vi "IDE_BT_Example.vi"() -> ()   [LabVIEW 2020]
uses:
  Subs/ColorText/Code.xctl
  Subs/Console XCtrl/Console_Xctrl.xctl
  Subs/Server XCtrl/Server.xctl
panel:
  in  "Files 2":bool
  in  "Open Server 2":bool
  in  "Help 2":bool
  in  "Name 2":string="code.py"
  in  "Save 2":bool
  in  "Stop 2":bool
  in  "Pyboard":string(xcontrol)="\n'''\nmac address of pybd: b'HJ0\\x01o\\xf2' or 48:4A:01:6F:F2\n    '''\n    '''\nHR_UUID = ubluetooth.UUID(0x180D)\nHR_CHAR = (ubluetooth.UUID(0x2A37), ubluetooth.FLAG_READ | ubluetooth.FLAG_NOTIFY,)\nHR_SERVICE = (HR_UUID, (HR_CHAR,),)\nSERVICES = (HR_SERVICE, )\n(hr,) = bt.gatts_register_services(SERVICES)\n'''\n\nimport bluetooth,utime\n\nble = bluetooth.BLE()\nble.active(True)\n\nLWP_CHAR = (\n    bluetooth.UUID('00001624-1212-EFDE-1623-785FEABCD123'),\n    bluetooth.FLAG_WRITE | bluetooth.FLAG_NOTIFY,\n    # List of descriptors\n    (\n        # CCCD\n        (bluetooth.UUID(0x2902), bluetooth.FLAG_READ | bluetooth.FLAG_WRITE),\n    )\n)\nLPF2_SERVICE = (bluetooth.UUID('03971101-0000-1000-8000-00805F9B34FB'), (LWP_CHAR,))\nALL_SERVICES = (LPF2_SERVICE,)\n\n(lwp_char, lwp_descr), = ble.gatts_register_services(ALL_SERVICES)\n\ndef bt_irq(x, y):\n    print('bt_irq', x, y)\n    \nble.irq(bt_irq)\n\ndef adv_encode_name(name):\n    name = bytes(name, 'ascii')\n    return bytearray((len(name) + 1, 0x09)) + name\n    \ndef adv(name):\n    ble.gap_advertise(100_000, adv_data=b'\\x02\\x01\\x06' + adv_encode_name(name))\n    \nadv('pybd-lpf2')\n\nutime.sleep(5)   # wait for pyboard to get ready and connect\n\nble.gatts_notify(64, lwp_char, 'from pybd')\n\nble.gatts_read(lwp_char)\n"
  in  "Run 2":bool
  in  "Clean 2":bool
  in  "PC Save 2":bool
  in  "PC path 2":path
  in  "Clear 2":bool
  out "REPL 2":string(xcontrol)="bt_irq', event, data)\n... \n... bt.irq(bt_irq, bluetooth.IRQ_ALL)\n... '''\n\"\\ndef bt_irq(event, data):\\n    print('bt_irq', event, data)\\n\\nbt.irq(bt_irq, bluetooth.IRQ_ALL)\\n\"\n>>> blurtooth.\nTraceback (most recent call last):\n  File \"<stdin>\", line 2\nSyntaxError: invalid syntax\n>>> bluetooth.\n__class__       __name__        BLE             FLAG_NOTIFY\nFLAG_READ       FLAG_WRITE      UUID\n>>> bt.\n__class__       active          config          gap_advertise\ngap_connect     gap_disconnect  gap_scan\ngattc_discover_characteristics  gattc_discover_descriptors\ngattc_discover_services         gattc_read      gattc_write\ngatts_notify    gatts_read      gatts_register_services\ngatts_set_buffer                gatts_write     irq\n>>> import bluetooth\n>>> bt = bluetooth.BLE()\n>>> bt.active(True)\nTrue\n>>> LPF2_SERVICE = bluetooth.UUID('00001623-1212-EFDE-1623-785FEABCD123')\n>>> LWP_CHAR = (bluetooth.UUID('00001624-1212-EFDE-1623-785FEABCD123'), bluetooth.FLAG_NOTIFY|bluetooth.FLAG_WRITE,)\n>>> lwp_char, = bt.gatts_register_services(LPF2_SERVICE, (LWP_CHAR,))\nTraceback (most recent call last):\n  File \"<stdin>\", line 1, in <module>\nTypeError: function takes 2 positional arguments but 3 were given\n>>> bt.gap_advertise(100, adv_data=bytearray('\\x02\\x01\\x02\\x0a\\x09pybd-lpf2'))\n>>> bt.gatts_notify(lwp_char, 64, 'from pybd')\nTraceback (most recent call last):\n  File \"<stdin>\", line 1, in <module>\nNameError: name 'lwp_char' isn't defined\n>>> bt.gatts_read(lwp_char)\nTraceback (most recent call last):\n  File \"<stdin>\", line 1, in <module>\nNameError: name 'lwp_char' isn't defined\n>>> '''\n... def bt_irq(event, data):\n...     print('bt_irq', event, data)\n... \n... bt.irq(bt_irq, bluetooth.IRQ_ALL)\n... '''\n\"\\ndef bt_irq(event, data):\\n    print('bt_irq', event, data)\\n\\nbt.irq(bt_irq, bluetooth.IRQ_ALL)\\n\"\n>>> '''\n... mac address of pybd: b'HJ0\\x01o\\xf2' or 48:4A:01:6F:F2\n... '''\n\"\\nmac address of pybd: b'HJ0\\x01o\\xf2' or 48:4A:01:6F:F2\\n\"\n>>> '''\n... \n... HR_UUID = ubluetooth.UUID(0x180D)\n... HR_CHAR = (ubluetooth.UUID(0x2A37), ubluetooth.FLAG_READ | ubluetooth.FLAG_NOTIFY,)\n... HR_SERVICE = (HR_UUID, (HR_CHAR,),)\n... SERVICES = (HR_SERVICE, )\n... (hr,) = bt.gatts_register_services(SERVICES)\n... '''\n'\\n\\nHR_UUID = ubluetooth.UUID(0x180D)\\nHR_CHAR = (ubluetooth.UUID(0x2A37), ubluetooth.FLAG_READ | ubluetooth.FLAG_NOTIFY,)\\nHR_SERVICE = (HR_UUID, (HR_CHAR,),)\\nSERVICES = (HR_SERVICE, )\\n(hr,) = bt.gatts_register_services(SERVICES)\\n'\n>>> import bluetooth,utime\n>>> ble = bluetooth.BLE()\n>>> ble.active(True)\nTrue\n>>> LWP_CHAR = (\n... bluetooth.UUID('00001624-1212-EFDE-1623-785FEABCD123'),\n... bluetooth.FLAG_WRITE | bluetooth.FLAG_NOTIFY,\n... (\n... (bluetooth.UUID(0x2902), bluetooth.FLAG_READ | bluetooth.FLAG_WRITE),\n... )\n... \n... )\n>>> LPF2_SERVICE = (bluetooth.UUID('00001623-1212-EFDE-1623-785FEABCD123'), (LWP_CHAR,))\n>>> ALL_SERVICES = (LPF2_SERVICE,)\n>>> (lwp_char, lwp_descr), = ble.gatts_register_services(ALL_SERVICES)\n>>> def bt_irq(x, y):\n...     print('bt_irq', x, y)\n... \n>>> ble.irq(bt_irq)\n>>> def adv_encode_name(name):\n...     name = bytes(name, 'ascii')\n...     return bytearray((len(name) + 1, 0x09)) + name\n... \n>>> def adv(name):\n...     ble.gap_advertise(100_000, adv_data=b'\\x02\\x01\\x06' + adv_encode_name(name))\n... \n>>> adv('pybd-lpf2')\n>>> utime.sleep(5)   \n>>> ble.gatts_notify(64, lwp_char, 'from pybd')\nTraceback (most recent call last):\n  File \"<stdin>\", line 1, in <module>\nOSError: [Errno 107] ENOTCONN\n>>> ble.gatts_read(lwp_char)\nb''\n>>> '''\n... mac address of pybd: b'HJ0\\x01o\\xf2' or 48:4A:01:6F:F2\n... '''\n\"\\nmac address of pybd: b'HJ0\\x01o\\xf2' or 48:4A:01:6F:F2\\n\"\n>>> '''\n... \n... HR_UUID = ubluetooth.UUID(0x180D)\n... HR_CHAR = (ubluetooth.UUID(0x2A37), ubluetooth.FLAG_READ | ubluetooth.FLAG_NOTIFY,)\n... HR_SERVICE = (HR_UUID, (HR_CHAR,),)\n... SERVICES = (HR_SERVICE, )\n... (hr,) = bt.gatts_register_services(SERVICES)\n... '''\n'\\n\\nHR_UUID = ubluetooth.UUID(0x180D)\\nHR_CHAR = (ubluetooth.UUID(0x2A37), ubluetooth.FLAG_READ | ubluetooth.FLAG_NOTIFY,)\\nHR_SERVICE = (HR_UUID, (HR_CHAR,),)\\nSERVICES = (HR_SERVICE, )\\n(hr,) = bt.gatts_register_services(SERVICES)\\n'\n>>> import bluetooth,utime\n>>> ble = bluetooth.BLE()\n>>> ble.active(True)\nTrue\n>>> LWP_CHAR = (\n... bluetooth.UUID('00001624-1212-EFDE-1623-785FEABCD123'),\n... bluetooth.FLAG_WRITE | bluetooth.FLAG_NOTIFY,\n... (\n... (bluetooth.UUID(0x2902), bluetooth.FLAG_READ | bluetooth.FLAG_WRITE),\n... )\n... \n... )\n>>> LPF2_SERVICE = (bluetooth.UUID('00001623-1212-EFDE-1623-785FEABCD123'), (LWP_CHAR,))\n>>> ALL_SERVICES = (LPF2_SERVICE,)\n>>> (lwp_char, lwp_descr), = ble.gatts_register_services(ALL_SERVICES)\n>>> def bt_irq(x, y):\n...     print('bt_irq', x, y)\n... \n>>> ble.irq(bt_irq)\n>>> def adv_encode_name(name):\n...     name = bytes(name, 'ascii')\n...     return bytearray((len(name) + 1, 0x09)) + name\n... \n>>> def adv(name):\n...     ble.gap_advertise(100_000, adv_data=b'\\x02\\x01\\x06' + adv_encode_name(name))\n... \n>>> adv('pybd-lpf2')\n>>> utime.sleep(5)   \n>>> ble.gatts_notify(64, lwp_char, 'from pybd')\nTraceback (most recent call last):\n  File \"<stdin>\", line 1, in <module>\nOSError: [Errno 107] ENOTCONN\n>>> ble.gatts_read(lwp_char)\nb''\n>>> '''\n... mac address of pybd: b'HJ0\\x01o\\xf2' or 48:4A:01:6F:F2\n... '''\n\"\\nmac address of pybd: b'HJ0\\x01o\\xf2' or 48:4A:01:6F:F2\\n\"\n>>> '''\n... \n... HR_UUID = ubluetooth.UUID(0x180D)\n... HR_CHAR = (ubluetooth.UUID(0x2A37), ubluetooth.FLAG_READ | ubluetooth.FLAG_NOTIFY,)\n... HR_SERVICE = (HR_UUID, (HR_CHAR,),)\n... SERVICES = (HR_SERVICE, )\n... (hr,) = bt.gatts_register_services(SERVICES)\n... '''\n'\\n\\nHR_UUID = ubluetooth.UUID(0x180D)\\nHR_CHAR = (ubluetooth.UUID(0x2A37), ubluetooth.FLAG_READ | ubluetooth.FLAG_NOTIFY,)\\nHR_SERVICE = (HR_UUID, (HR_CHAR,),)\\nSERVICES = (HR_SERVICE, )\\n(hr,) = bt.gatts_register_services(SERVICES)\\n'\n>>> import bluetooth,utime\n>>> ble = bluetooth.BLE()\n>>> ble.active(True)\nTrue\n>>> LWP_CHAR = (\n... bluetooth.UUID('00001624-1212-EFDE-1623-785FEABCD123'),\n... bluetooth.FLAG_WRITE | bluetooth.FLAG_NOTIFY,\n... (\n... (bluetooth.UUID(0x2902), bluetooth.FLAG_READ | bluetooth.FLAG_WRITE),\n... )\n... \n... )\n>>> LPF2_SERVICE = (bluetooth.UUID('03971101-0000-1000-8000-00805F9B34FB'), (LWP_CHAR,))\n>>> ALL_SERVICES = (LPF2_SERVICE,)\n>>> (lwp_char, lwp_descr), = ble.gatts_register_services(ALL_SERVICES)\n>>> def bt_irq(x, y):\n...     print('bt_irq', x, y)\n... \n>>> ble.irq(bt_irq)\n>>> def adv_encode_name(name):\n...     name = bytes(name, 'ascii')\n...     return bytearray((len(name) + 1, 0x09)) + name\n... \n>>> def adv(name):\n...     ble.gap_advertise(100_000, adv_data=b'\\x02\\x01\\x06' + adv_encode_name(name))\n... \n>>> adv('pybd-lpf2')\n>>> utime.sleep(5)   \n>>> ble.gatts_notify(64, lwp_char, 'from pybd')\nTraceback (most recent call last):\n  File \"<stdin>\", line 1, in <module>\nOSError: [Errno 107] ENOTCONN\n>>> ble.gatts_read(lwp_char)\nb''\n>>> \nMPY: sync filesystems\nMPY: soft reboot\nMicroPython v1.11-611-g7f24c2977-dirty on 2019-11-29; PYBD-SF2W with STM32F722IEK\nType \"help()\" for more information.\n>>> '''\n... mac address of pybd: b'HJ0\\x01o\\xf2' or 48:4A:01:6F:F2\n... '''\n\"\\nmac address of pybd: b'HJ0\\x01o\\xf2' or 48:4A:01:6F:F2\\n\"\n>>> '''\n... \n... HR_UUID = ubluetooth.UUID(0x180D)\n... HR_CHAR = (ubluetooth.UUID(0x2A37), ubluetooth.FLAG_READ | ubluetooth.FLAG_NOTIFY,)\n... HR_SERVICE = (HR_UUID, (HR_CHAR,),)\n... SERVICES = (HR_SERVICE, )\n... (hr,) = bt.gatts_register_services(SERVICES)\n... '''\n'\\n\\nHR_UUID = ubluetooth.UUID(0x180D)\\nHR_CHAR = (ubluetooth.UUID(0x2A37), ubluetooth.FLAG_READ | ubluetooth.FLAG_NOTIFY,)\\nHR_SERVICE = (HR_UUID, (HR_CHAR,),)\\nSERVICES = (HR_SERVICE, )\\n(hr,) = bt.gatts_register_services(SERVICES)\\n'\n>>> import bluetooth,utime\n>>> ble = bluetooth.BLE()\n>>> ble.active(True)\nTrue\n>>> LWP_CHAR = (\n... bluetooth.UUID('00001624-1212-EFDE-1623-785FEABCD123'),\n... bluetooth.FLAG_WRITE | bluetooth.FLAG_NOTIFY,\n... (\n... (bluetooth.UUID(0x2902), bluetooth.FLAG_READ | bluetooth.FLAG_WRITE),\n... )\n... \n... )\n>>> LPF2_SERVICE = (bluetooth.UUID('03971101-0000-1000-8000-00805F9B34FB'), (LWP_CHAR,))\n>>> ALL_SERVICES = (LPF2_SERVICE,)\n>>> (lwp_char, lwp_descr), = ble.gatts_register_services(ALL_SERVICES)\n>>> def bt_irq(x, y):\n...     print('bt_irq', x, y)\n... \n>>> ble.irq(bt_irq)\n>>> def adv_encode_name(name):\n...     name = bytes(name, 'ascii')\n...     return bytearray((len(name) + 1, 0x09)) + name\n... \n>>> def adv(name):\n...     ble.gap_advertise(100_000, adv_data=b'\\x02\\x01\\x06' + adv_encode_name(name))\n... \n>>> adv('pybd-lpf2')\n>>> utime.sleep(5)   \n>>> ble.gatts_notify(64, lwp_char, 'from pybd')\nTraceback (most recent call last):\n  File \"<stdin>\", line 1, in <module>\nOSError: [Errno 107] ENOTCONN\n>>> ble.gatts_read(lwp_char)\nb''\n>>> bt_irq 1 (64, 1, b\"N'\\xee\\xa63)\")\nbt_irq 4 (64, 13)\nbt_irq 4 (64, 13)\n\n>>> ble.gatts_read(lwp_char)\nb'\\xff'\n>>> bt_irq 4 (64, 13)\n\n>>> ble.gatts_read(lwp_char)\nb'z'\n>>> ble.\n__class__       active          config          gap_advertise\ngap_connect     gap_disconnect  gap_scan\ngattc_discover_characteristics  gattc_discover_descriptors\ngattc_discover_services         gattc_read      gattc_write\ngatts_notify    gatts_read      gatts_register_services\ngatts_set_buffer                gatts_write     irq\n>>> bluetooth.\n__class__       __name__        BLE             FLAG_NOTIFY\nFLAG_READ       FLAG_WRITE      UUID\n>>> bluetooth.UUID()\nTraceback (most recent call last):\n  File \"<stdin>\", line 1, in <module>\nTypeError: function takes 1 positional arguments but 0 were given\n>>> \n>>> bt_irq 2 (64, 1, b\"N'\\xee\\xa63)\")\n\n>>> bluetooth.\n__class__       __name__        BLE             FLAG_NOTIFY\nFLAG_READ       FLAG_WRITE      UUID\n>>> bluetooth.BLE.\n__class__       __name__        __bases__       active\nconfig          gap_advertise   gap_connect     gap_disconnect\ngap_scan        gattc_discover_characteristics\ngattc_discover_descriptors      gattc_discover_services\ngattc_read      gattc_write     gatts_notify    gatts_read\ngatts_register_services         gatts_set_buffer\ngatts_write     irq\n>>> bluetooth.BLE."
  in  "Server 2":path(xcontrol)=path "/Users/crogers/GitHub/Summer2020/LabVIEWCode/Servers/Damien.vi"
  in  "Clean":bool
  in  "PC Save":bool
  in  "PC path":path
  in  "Files":bool
  in  "Open Server":bool
  in  "Help":bool
  in  "Server":path(xcontrol)=path "/Users/crogers/GitHub/Summer2020/LabVIEWCode/Servers/Jens.vi"
  out "REPL":string(xcontrol)="p\":[[0, []], [0, []], [0, []], [0, []], [0, []], [0, []], [-31, 30, 995], [2, 5, 1], [8, 1, -1], \"\", 0]}{\"m\":0,\"p\":[[0, []], [0, []], [0, []], [0, []], [0, []], [0, []], [-30, 27, 991], [3, 5, 1], [8, 1, -1], \"\", 0]}{\"m\":0,\"p\":[[0, []], [0, []], [0, []], [0, []], [0, []], [0, []], [-29, 26, 993], [2, 5, 1], [8, 1, -1], \"\", 0]}{\"m\":0,\"p\":[[0, []], [0, []], [0, []], [0, []], [0, []], [0, []], [-29, 28, 992], [3, 5, 0], [8, 1, -1], \"\", 0]}{\"m\":0,\"p\":[[0, []], [0, []], [0, []], [0, []], [0, []], [0, []], [-29, 28, 990], [3, 5, 1], [8, 1, -1], \"\", 0]}{\"m\":0,\"p\":[[0, []], [0, []], [0, []], [0, []], [0, []], [0, []], [-29, 27, 994], [2, 5, 1], [8, 1, -1], \"\", 0]}{\"m\":0,\"p\":[[0, []], [0, []], [0, []], [0, []], [0, []], [0, []], [-29, 30, 991], [3, 5, 1], [8, 1, -1], \"\", 0]}{\"m\":0,\"p\":[[0, []], [0, []], [0, []], [0, []], [0, []], [0, []], [-27, 27, 993], [3, 5, 1], [8, 1, -1], \"\", 0]}{\"m\":0,\"p\":[[0, []], [0, []], [0, []], [0, []], [0, []], [0, []], [-29, 28, 992], [2, 4, 1], [8, 1, -1], \"\", 0]}{\"m\":0,\"p\":[[0, []], [0, []], [0, []], [0, []], [0, []], [0, []], [-29, 28, 989], [2, 5, 1], [8, 1, -1], \"\", 0]}{\"m\":0,\"p\":[[0, []], [0, []], [0, []], [0, []], [0, []], [0, []], [-28, 28, 989], [2, 5, 1], [8, 1, -1], \"\", 0]}{\"m\":0,\"p\":[[0, []], [0, []], [0, []], [0, []], [0, []], [0, []], [-28, 29, 992], [3, 5, 1], [8, 1, -1], \"\", 0]}{\"m\":0,\"p\":[[0, []], [0, []], [0, []], [0, []], [0, []], [0, []], [-28, 28, 993], [3, 5, 0], [8, 1, -1], \"\", 0]}{\"m\":0,\"p\":[[0, []], [0, []], [0, []], [0, []], [0, []], [0, []], [-29, 29, 993], [2, 4, 1], [8, 1, -1], \"\", 0]}{\"m\":0,\"p\":[[0, []], [0, []], [0, []], [0, []], [0, []], [0, []], [-28, 28, 992], [2, 5, 1], [8, 1, -1], \"\", 0]}{\"m\":2,\"p\":[8.357, 100]}{\"m\":0,\"p\":[[0, []], [0, []], [0, []], [0, []], [0, []], [0, []], [-31, 31, 991], [2, 5, 1], [8, 1, -1], \"\", 0]}{\"m\":0,\"p\":[[0, []], [0, []], [0, []], [0, []], [0, []], [0, []], [-31, 30, 994], [2, 5, 1], [8, 1, -1], \"\", 0]}{\"m\":0,\"p\":[[0, []], [0, []], [0, []], [0, []], [0, []], [0, []], [-28, 28, 992], [3, 4, 1], [8, 1, -1], \"\", 0]}{\"m\":0,\"p\":[[0, []], [0, []], [0, []], [0, []], [0, []], [0, []], [-29, 28, 993], [2, 5, 1], [8, 1, -1], \"\", 0]}{\"m\":0,\"p\":[[0, []], [0, []], [0, []], [0, []], [0, []], [0, []], [-30, 28, 991], [3, 5, 0], [8, 1, -1], \"\", 0]}{\"m\":0,\"p\":[[0, []], [0, []], [0, []], [0, []], [0, []], [0, []], [-30, 29, 994], [3, 5, 1], [8, 1, -1], \"\", 0]}{\"m\":0,\"p\":[[0, []], [0, []], [0, []], [0, []], [0, []], [0, []], [-29, 29, 992], [2, 4, 1], [8, 1, -1], \"\", 0]}{\"m\":0,\"p\":[[0, []], [0, []], [0, []], [0, []], [0, []], [0, []], [-30, 27, 990], [2, 5, 1], [8, 1, -1], \"\", 0]}{\"m\":0,\"p\":[[0, []], [0, []], [0, []], [0, []], [0, []], [0, []], [-29, 28, 992], [2, 5, 1], [8, 1, -1], \"\", 0]}{\"m\":0,\"p\":[[0, []], [0, []], [0, []], [0, []], [0, []], [0, []], [-32, 31, 993], [2, 5, 1], [8, 1, -1], \"\", 0]}{\"m\":0,\"p\":[[0, []], [0, []], [0, []], [0, []], [0, []], [0, []], [-29, 28, 992], [2, 5, 1], [8, 1, -1], \"\", 0]}{\"m\":0,\"p\":[[0, []], [0, []], [0, []], [0, []], [0, []], [0, []], [-31, 29, 989], [2, 5, 1], [8, 1, -1], \"\", 0]}{\"m\":0,\"p\":[[0, []], [0, []], [0, []], [0, []], [0, []], [0, []], [-30, 27, 993], [3, 5, 1], [8, 1, -1], \"\", 0]}{\"m\":0,\"p\":[[0, []], [0, []], [0, []], [0, []], [0, []], [0, []], [-31, 28, 993], [3, 5, 1], [8, 1, -1], \"\", 0]}{\"m\":0,\"p\":[[0, []], [0, []], [0, []], [0, []], [0, []], [0, []], [-31, 27, 994], [3, 5, 0], [8, 1, -1], \"\", 0]}{\"m\":0,\"p\":[[0, []], [0, []], [0, []], [0, []], [0, []], [0, []], [-31, 26, 994], [3, 4, 1], [8, 1, -1], \"\", 0]}{\"m\":0,\"p\":[[0, []], [0, []], [0, []], [0, []], [0, []], [0, []], [-29, 28, 991], [3, 4, 0], [8, 1, -1], \"\", 0]}{\"m\":0,\"p\":[[0, []], [0, []], [0, []], [0, []], [0, []], [0, []], [-29, 27, 990], [2, 5, 1], [8, 1, -1], \"\", 0]}{\"m\":0,\"p\":[[0, []], [0, []], [0, []], [0, []], [0, []], [0, []], [-28, 27, 990], [3, 5, 1], [8, 1, -1], \"\", 0]}{\"m\":0,\"p\":[[0, []], [0, []], [0, []], [0, []], [0, []], [0, []], [-30, 28, 991], [3, 5, 1], [8, 1, -1], \"\", 0]}{\"m\":2,\"p\":[8.36, 100]}{\"m\":0,\"p\":[[0, []], [0, []], [0, []], [0, []], [0, []], [0, []], [-29, 27, 992], [3, 5, 1], [8, 1, -1], \"\", 0]}{\"m\":0,\"p\":[[0, []], [0, []], [0, []], [0, []], [0, []], [0, []], [-29, 28, 994], [2, 5, 0], [8, 1, -1], \"\", 0]}{\"m\":0,\"p\":[[0, []], [0, []], [0, []], [0, []], [0, []], [0, []], [-29, 27, 993], [2, 5, 1], [8, 1, -1], \"\", 0]}{\"m\":0,\"p\":[[0, []], [0, []], [0, []], [0, []], [0, []], [0, []], [-30, 28, 994], [3, 5, 0], [8, 1, -1], \"\", 0]}{\"m\":0,\"p\":[[0, []], [0, []], [0, []], [0, []], [0, []], [0, []], [-29, 29, 992], [2, 5, 1], [8, 1, -1], \"\", 0]}{\"m\":0,\"p\":[[0, []], [0, []], [0, []], [0, []], [0, []], [0, []], [-31, 29, 994], [3, 5, 0], [8, 1, -1], \"\", 0]}{\"m\":0,\"p\":[[0, []], [0, []], [0, []], [0, []], [0, []], [0, []], [-28, 29, 991], [3, 4, 1], [8, 1, -1], \"\", 0]}{\"m\":0,\"p\":[[0, []], [0, []], [0, []], [0, []], [0, []], [0, []], [-29, 31, 992], [2, 5, 0], [8, 1, -1], \"\", 0]}{\"m\":0,\"p\":[[0, []], [0, []], [0, []], [0, []], [0, []], [0, []], [-31, 27, 992], [3, 5, 1], [8, 1, -1], \"\", 0]}{\"m\":0,\"p\":[[0, []], [0, []], [0, []], [0, []], [0, []], [0, []], [-29, 28, 994], [2, 4, 0], [8, 1, -1], \"\", 0]}{\"m\":0,\"p\":[[0, []], [0, []], [0, []], [0, []], [0, []], [0, []], [-30, 29, 994], [2, 5, 1], [8, 1, -1], \"\", 0]}{\"m\":0,\"p\":[[0, []], [0, []], [0, []], [0, []], [0, []], [0, []], [-28, 30, 992], [2, 4, 1], [8, 1, -1], \"\", 0]}{\"m\":0,\"p\":[[0, []], [0, []], [0, []], [0, []], [0, []], [0, []], [-29, 28, 990], [2, 5, 1], [8, 1, -1], \"\", 0]}{\"m\":0,\"p\":[[0, []], [0, []], [0, []], [0, []], [0, []], [0, []], [-28, 29, 996], [3, 5, 1], [8, 1, -1], \"\", 0]}{\"m\":0,\"p\":[[0, []], [0, []], [0, []], [0, []], [0, []], [0, []], [-28, 26, 994], [2, 4, 1], [8, 1, -1], \"\", 0]}{\"m\":0,\"p\":[[0, []], [0, []], [0, []], [0, []], [0, []], [0, []], [-28, 28, 991], [2, 4, 1], [8, 1, -1], \"\", 0]}{\"m\":0,\"p\":[[0, []], [0, []], [0, []], [0, []], [0, []], [0, []], [-28, 27, 992], [3, 5, 1], [8, 1, -1], \"\", 0]}{\"m\":0,\"p\":[[0, []], [0, []], [0, []], [0, []], [0, []], [0, []], [-30, 27, 994], [2, 5, 1], [8, 1, -1], \"\", 0]}{\"m\":0,\"p\":[[0, []], [0, []], [0, []], [0, []], [0, []], [0, []], [-29, 28, 989], [2, 4, 1], [8, 1, -1], \"\", 0]}{\"m\":0,\"p\":[[0, []], [0, []], [0, []], [0, []], [0, []], [0, []], [-28, 29, 991], [2, 5, 1], [8, 1, -1], \"\", 0]}{\"m\":2,\"p\":[8.357, 100]}{\"m\":0,\"p\":[[0, []], [0, []], [0, []], [0, []], [0, []], [0, []], [-28, 28, 994], [2, 5, 0], [8, 1, -1], \"\", 0]}{\"m\":0,\"p\":[[0, []], [0, []], [0, []], [0, []], [0, []], [0, []], [-29, 29, 991], [2, 4, 1], [8, 1, -1], \"\", 0]}Traceback (most recent call last):\n  File \"main.py\", line 8, in <module>\n  File \"lib/hub/flash/hub_runtime.py\", line 1, in start\nKeyboardInterrupt: \nMicroPython v1.10-1531-ge24b9b97f on 2020-05-06; LEGO Technic Large Hub with STM32F413xx\nType \"help()\" for more information.\n>>> import hub,utime\n>>> hub.bluetooth.info()\n{'mac_addr': '40:BD:32:41:4F:A3', 'service_uuid': '03971101-0000-1000-8000-00805F9B34FB', 'name': 'LEGO Hub@HomeHub', 'iap': {'device_version': 7, 'authentication_revision': 1, 'device_id': '00:00:03:00', 'certificate_serial_no': '542F24F6FE7C713FF69C1D500590FF35', 'protocol_major_version': 3, 'protocol_minor_version': 0}, 'known_devices': ['F0:18:98:55:52:74', 'DC:A9:04:96:70:29'], 'device_uuid': '03970000-3800-2100-0951-383138393536'}\n>>> def FindIt():\n...     hub.ble.scan (5)\n...     board = -1\n...     while board < 0:\n...         utime.sleep_ms(100)\n...         clients = hub.ble.scan_result()\n...         i=0\n...         for client in clients:\n...             if client['mac_addr'] ==  '48:4A:30:01:98:62':\n...                 print(\"found it\")\n...                 board = i\n...                 break\n...             i += 1\n...     return board\n... \n>>> board = Findit()\nTraceback (most recent call last):\n  File \"<stdin>\", line 1, in <module>\nNameError: name 'Findit' isn't defined\n>>> if (board > 0):\n...     p = hub.ble.connect(board)\n...     if p:\n...         p_info = p.info()\n...         print(p_info)\n...         p.callback(lambda v: print('got data:', v))\n...         p.subscribe()\n...         p.send('from hub')\n...         utime.sleep(10)\n...         p.unsubscribe()\n...         p.disconnect(p_info['index'])\n...         \n...         \n... \nTraceback (most recent call last):\n  File \"<stdin>\", line 1, in <module>\nNameError: name 'board' isn't defined\n>>> FindIt()\nTraceback (most recent call last):\n  File \"<stdin>\", line 1, in <module>\n  File \"<stdin>\", line 5, in FindIt\nKeyboardInterrupt: \n>>> import hub,utime\n>>> hub.bluetooth.info()\n{'mac_addr': '40:BD:32:41:4F:A3', 'service_uuid': '03971101-0000-1000-8000-00805F9B34FB', 'name': 'LEGO Hub@HomeHub', 'iap': {'device_version': 7, 'authentication_revision': 1, 'device_id': '00:00:03:00', 'certificate_serial_no': '542F24F6FE7C713FF69C1D500590FF35', 'protocol_major_version': 3, 'protocol_minor_version': 0}, 'known_devices': ['F0:18:98:55:52:74', 'DC:A9:04:96:70:29'], 'device_uuid': '03970000-3800-2100-0951-383138393536'}\n>>> def FindIt():\n...     hub.ble.scan (5)\n...     board = -1\n...     while board < 0:\n...         utime.sleep_ms(100)\n...         clients = hub.ble.scan_result()\n...         i=0\n...         for client in clients:\n...             if client['mac_addr'] ==  '48:4A:30:01:98:62':\n...                 print(\"found it\")\n...                 board = i\n...                 break\n...             i += 1\n...     return board\n... \n>>> board = FindIt()\n{\"m\":4,\"p\":\"doubletapped\"}Traceback (most recent call last):\n  File \"<stdin>\", line 1, in <module>\n  File \"<stdin>\", line 5, in FindIt\nKeyboardInterrupt: \n>>> if (board > 0):\n...     p = hub.ble.connect(board)\n...     if p:\n...         p_info = p.info()\n...         print(p_info)\n...         p.callback(lambda v: print('got data:', v))\n...         p.subscribe()\n...         p.send('from hub')\n...         utime.sleep(10)\n...         p.unsubscribe()\n...         p.disconnect(p_info['index'])\n...         \n...         \n... \nTraceback (most recent call last):\n  File \"<stdin>\", line 1, in <module>\nNameError: name 'board' isn't defined\n>>> {\"m\":3,\"p\":[\"connect\", 0]}{\"m\":3,\"p\":[\"connect\", 130]}"
  in  "Clear":bool
  in  "Save":bool
  in  "Stop":bool
  in  "Run":bool
  in  "Name":string="code.py"
  in  "SPIKE Prime":string(xcontrol)="import hub,utime\n\nhub.bluetooth.info()\n\ndef FindIt():\n    hub.ble.scan (5)\n    \n    board = -1\n    while board < 0:\n        utime.sleep_ms(100)\n        clients = hub.ble.scan_result()\n#     print(len(clients))\n        i=0\n        for client in clients:\n#               if client['service_id'] ==  '14200126-D700-0032-6670-6C2D64627970':\n                if client['mac_addr'] ==  '48:4A:30:01:98:62':\n                    print(\"found it\")\n                    board = i\n                    break\n                i += 1\n        return board\n        \nboard = FindIt()\n#print(board)\n\nif (board > 0):\n    p = hub.ble.connect(board)\n    if p:\n        p_info = p.info()\n        print(p_info)\n        p.callback(lambda v: print('got data:', v))\n        p.subscribe()\n        \n        p.send('from hub')\n        \n        utime.sleep(10)\n        p.unsubscribe()\n        p.disconnect(p_info['index'])\n        \n        \n        \n        \n        \n        \n        "
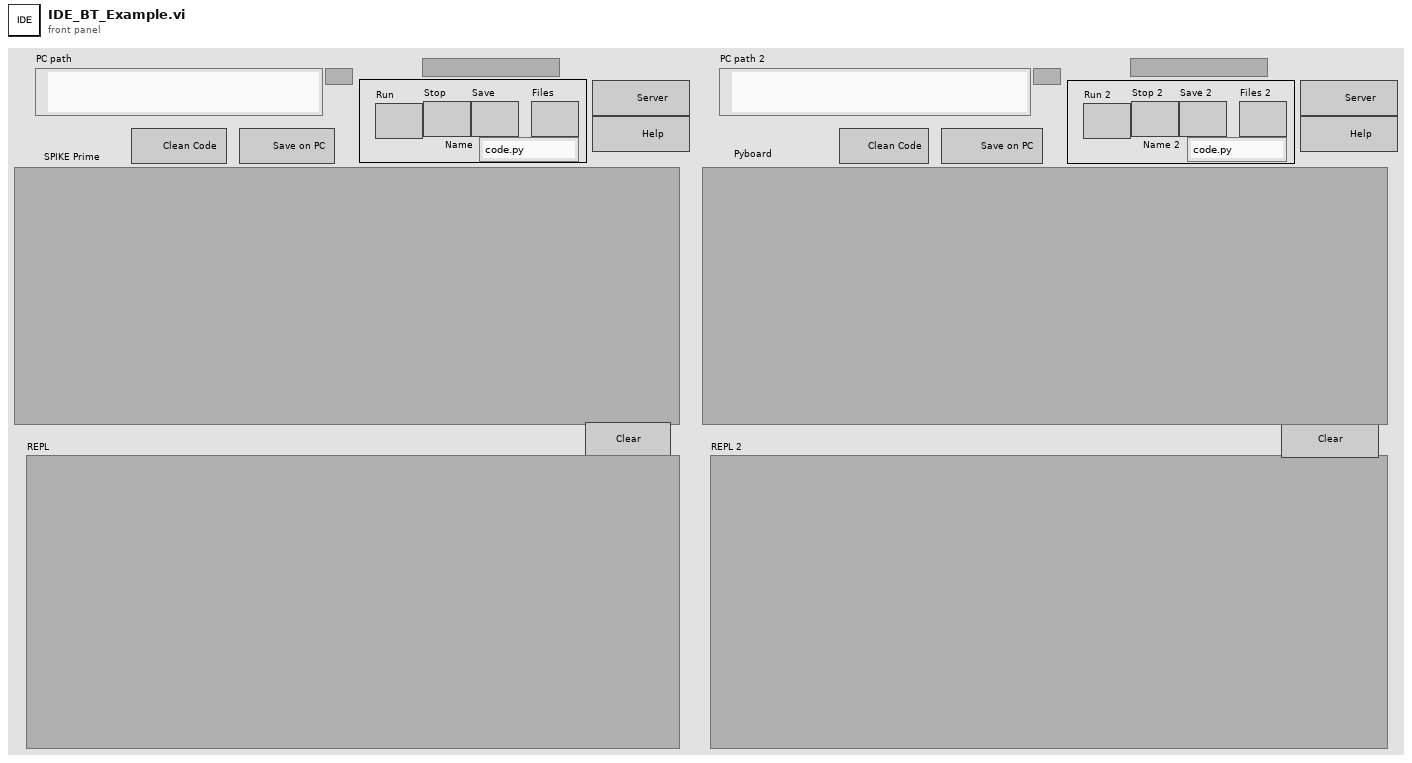
[diagram p1: front panel]
types:
  T1 = cluster{"Quote":u32, "Comment":u32, "Python":u32, "Text":u32, "Triple Quote":u32, "function":u32, "Line numbers":u32, "REPL Err":u32, "REPL Text":u32, "Text Bkgd":u32, "REPL Bkgd":u32}
  T2 = enum8{"Enabled", "Disabled", "Disabled and Grayed Out"}
  T3 = typedef "eventvkey.ctl" = enum16{"ASCII", "Enter", "Return", "Shift", "Ctrl", "Alt", "Cmd", "Opt", "Caps", "NumLock", "Clear", "Break", "Up", "Down", "Left", "Right", "Insert", "Delete", "Home", "End", "PageUp", "PageDown", "Escape", "Help", "Pause", "ScrollLock", "F1", "F2", "F3", "F4", "F5", "F6", "F7", "F8", "F9", "F10", "F11", "F12", "F13", "F14", "F15", "F16", "F17", "F18", "F19", "F20", "F21", "F22", "F23", "F24", "Play", "VolumeUp", "VolumeDown", "Mute", "Two Byte Char"}
  T4 = cluster{"Shift":bool, "Ctrl":bool, "Alt":bool, "Cmd":bool, "Opt":bool}
  T5 = cluster{"Char":i16, "VKey":T3, "PlatMods":cluster{"Shift":bool, "Ctrl":bool, "Alt":bool, "Cmd":bool, "Opt":bool}}
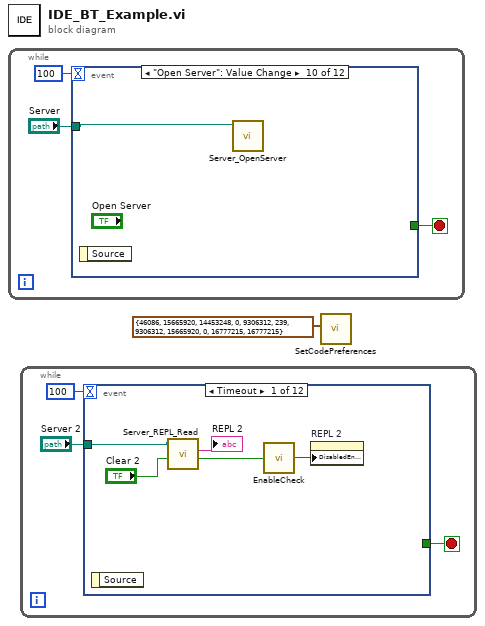
[diagram p0: block diagram]
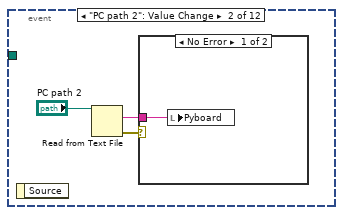
[diagram p2: hidden frame]
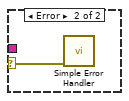
[diagram p3: hidden frame]
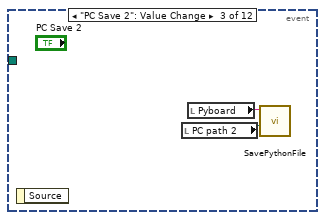
[diagram p4: hidden frame]
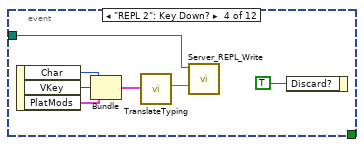
[diagram p5: hidden frame]
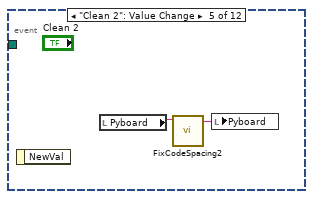
[diagram p6: hidden frame]
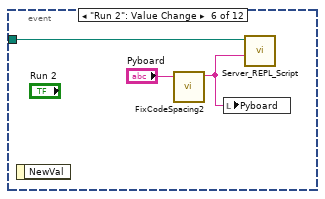
[diagram p7: hidden frame]
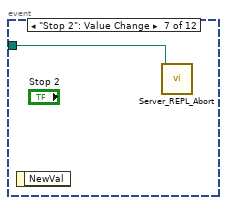
[diagram p8: hidden frame]
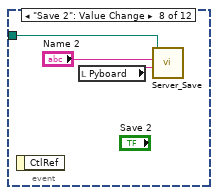
[diagram p9: hidden frame]
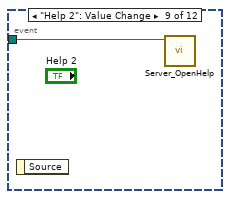
[diagram p10: hidden frame]
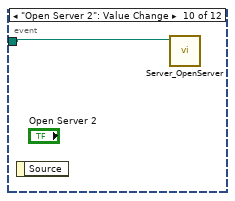
[diagram p11: hidden frame]
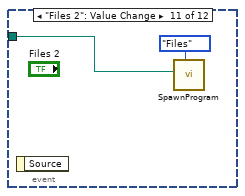
[diagram p12: hidden frame]
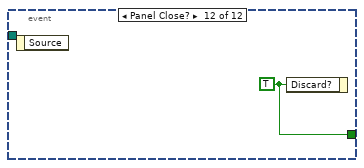
[diagram p13: hidden frame]
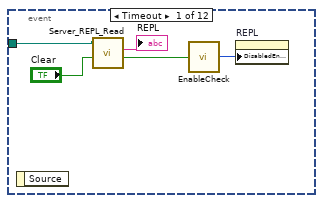
[diagram p14: hidden frame]
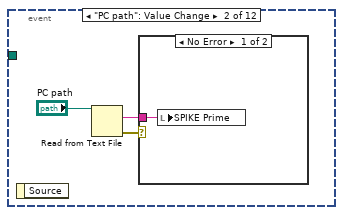
[diagram p15: hidden frame]
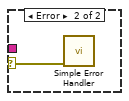
[diagram p16: hidden frame]
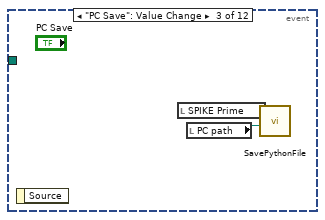
[diagram p17: hidden frame]
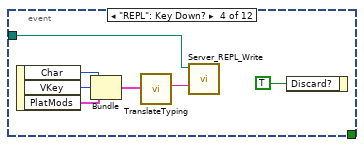
[diagram p18: hidden frame]
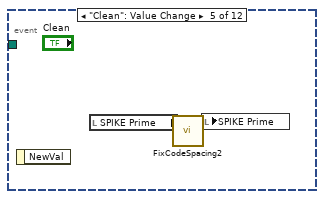
[diagram p19: hidden frame]
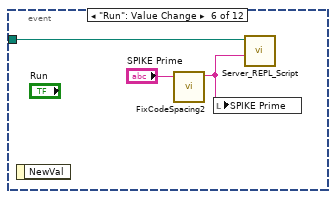
[diagram p20: hidden frame]
diagram:
  n1 = while {
    stop <- w3 stop-if-true
    n2 = event shown="[9] \"Open Server\": Value Change" {
      selector: _ -> [_ _ _ _ _ _ _ _ _ _ _ _]
      dyn-events: _ -> [_ _ _ _ _ _ _ _ _ _ _ _]
      timeout: 100 -> [_ _ _ _ _ _ _ _ _ _ _ _]
      tunnel: [_ _ _ _ _ _ _ _ _ _ _ w37] -> w3
      tunnel: "Server" -> [w7 _ _ w17 _ w27 w29 w30 w33 w34 w36 _]
      event Timeout {
        n3 = event-data() -> ()  [unwired: 1 in, 1 out]
        n4 = call "Server_REPL_Read.vi"("Clear"="Clear", "Server"=w7) -> ("Running?"=w8:bool, "REPL"=→"REPL":string)  [unwired: 7 in, 1 out]
        n5 = call "EnableCheck.vi"("Enable?"=w8) -> ("Enum"=w9:T2)
        n6 = property on="REPL" class="Console_Xctrl (strict)"("DisabledEnum"=w9) -> ()  [unwired: 2 in, 2 out]
      }
      event "PC path": Value Change {
        n7 = event-data() -> ()  [unwired: 1 in, 1 out]
        n8 = Read from Text File(file (use dialog)="PC path") -> (text=w11:string, error out=w12:errorcluster)  [unwired: 3 in, 2 out]
        n9 = case shown="No Error" w12 {
          selector: w12 -> [_ w14]
          tunnel: w11 -> [w13 _]
          frame No Error {
            n10 = local write "SPIKE Prime"(w13) -> ()
          }
          frame Error {
            n11 = call <vilib>:"Simple Error Handler.vi"("error in (no error)"=w14) -> ()  [unwired: 4 in, 5 out]
          }
        }
      }
      event "PC Save": Value Change {
        n12 = event-data() -> ()  [unwired: 1 in, 1 out]
        n13 = local read "SPIKE Prime"() -> (w16:string)
        n14 = local read "PC path"() -> (w15:path)
        n15 = call "SavePythonFile.vi"("path"=w15, "Code"=w16) -> ()  [unwired: 10 in]
      }
      event "REPL": Key Down? {
        n16 = event-data() -> ("Char"=w22:i16, "VKey"=w21:T3, "PlatMods"=w19:T4)  [unwired: 1 in]
        n17 = Bundle("Char"=w22, "VKey"=w21, "PlatMods"=w19) -> (w23:T5)  [unwired: 1 in]
        n18 = call "TranslateTyping.vi"("Cluster"=w23) -> ("key"=w18:string)  [unwired: 10 in]
        n19 = call "Server_REPL_Write.vi"("Code"=w18, "Server"=w17) -> ()  [unwired: 9 in, 1 out]
        n20 = event-data("Discard?"=TRUE) -> ()  [unwired: 1 in, 1 out]
      }
      event "Clean": Value Change {
        n21 = event-data() -> ()  [unwired: 1 in, 1 out]
        n22 = local read "SPIKE Prime"() -> (w24:string)
        n23 = call "FixCodeSpacing2.vi"("Code"=w24) -> ("Cleaned"=w25:string)  [unwired: 10 in]
        n24 = local write "SPIKE Prime"(w25) -> ()
      }
      event "Run": Value Change {
        n25 = event-data() -> ()  [unwired: 1 in, 1 out]
        n26 = call "FixCodeSpacing2.vi"("Code"="SPIKE Prime") -> ("Cleaned"=w26:string)  [unwired: 10 in]
        n27 = local write "SPIKE Prime"(w26) -> ()
        n28 = call "Server_REPL_Script.vi"("Code"=w26, "Server"=w27) -> ()  [unwired: 9 in, 1 out]
      }
      event "Stop": Value Change {
        n29 = event-data() -> ()  [unwired: 1 in, 1 out]
        n30 = call "Server_REPL_Abort.vi"("Server"=w29) -> ()  [unwired: 10 in, 1 out]
      }
      event "Save": Value Change {
        n31 = event-data() -> ()  [unwired: 1 in, 1 out]
        n32 = local read "SPIKE Prime"() -> (w32:string)
        n33 = call "Server_Save.vi"("Code"=w32, "Name"="Name", "Server"=w30) -> ()  [unwired: 8 in, 1 out]
      }
      event "Help": Value Change {
        n34 = event-data() -> ()  [unwired: 1 in, 1 out]
        n35 = call "Server_OpenHelp.vi"("Server"=w33) -> ()  [unwired: 10 in, 1 out]
      }
      event "Open Server": Value Change {
        n36 = event-data() -> ()  [unwired: 1 in, 1 out]
        n37 = call "Server_OpenServer.vi"("Server"=w34) -> ()  [unwired: 10 in, 1 out]
      }
      event "Files": Value Change {
        n38 = event-data() -> ()  [unwired: 1 in, 1 out]
        n39 = call "SpawnProgram.vi"("Server"=w36, "Dialog"=enum16{"Help", "Files"}."Files") -> ()  [unwired: 10 in]
      }
      event Panel Close? {
        w37 = TRUE ("Discard?")
        n40 = event-data() -> ()  [unwired: 1 in, 1 out]
        n41 = event-data("Discard?"=w37) -> ()  [unwired: 1 in, 1 out]
      }
    }
  }
  n42 = while {
    stop <- w39 stop-if-true
    n43 = event shown="[0] Timeout" {
      selector: _ -> [_ _ _ _ _ _ _ _ _ _ _ _]
      dyn-events: _ -> [_ _ _ _ _ _ _ _ _ _ _ _]
      timeout: 100 -> [_ _ _ _ _ _ _ _ _ _ _ _]
      tunnel: [_ _ _ _ _ _ _ _ _ _ _ w73] -> w39
      tunnel: "Server 2" -> [w43 _ _ w53 _ w63 w65 w66 w69 w70 w72 _]
      event Timeout {
        n44 = event-data() -> ()  [unwired: 1 in, 1 out]
        n45 = call "Server_REPL_Read.vi"("Clear"="Clear 2", "Server"=w43) -> ("Running?"=w44:bool, "REPL"=→"REPL 2":string)  [unwired: 7 in, 1 out]
        n46 = call "EnableCheck.vi"("Enable?"=w44) -> ("Enum"=w45:T2)
        n47 = property on="REPL 2" class="Console_Xctrl (strict)"("DisabledEnum"=w45) -> ()  [unwired: 2 in, 2 out]
      }
      event "PC path 2": Value Change {
        n48 = event-data() -> ()  [unwired: 1 in, 1 out]
        n49 = Read from Text File(file (use dialog)="PC path 2") -> (text=w47:string, error out=w48:errorcluster)  [unwired: 3 in, 2 out]
        n50 = case shown="No Error" w48 {
          selector: w48 -> [_ w50]
          tunnel: w47 -> [w49 _]
          frame No Error {
            n51 = local write "Pyboard"(w49) -> ()
          }
          frame Error {
            n52 = call <vilib>:"Simple Error Handler.vi"("error in (no error)"=w50) -> ()  [unwired: 4 in, 5 out]
          }
        }
      }
      event "PC Save 2": Value Change {
        n53 = event-data() -> ()  [unwired: 1 in, 1 out]
        n54 = local read "PC path 2"() -> (w51:path)
        n55 = local read "Pyboard"() -> (w52:string)
        n56 = call "SavePythonFile.vi"("path"=w51, "Code"=w52) -> ()  [unwired: 10 in]
      }
      event "REPL 2": Key Down? {
        n57 = event-data() -> ("Char"=w58:i16, "VKey"=w57:T3, "PlatMods"=w55:T4)  [unwired: 1 in]
        n58 = Bundle("Char"=w58, "VKey"=w57, "PlatMods"=w55) -> (w59:T5)  [unwired: 1 in]
        n59 = call "TranslateTyping.vi"("Cluster"=w59) -> ("key"=w54:string)  [unwired: 10 in]
        n60 = call "Server_REPL_Write.vi"("Code"=w54, "Server"=w53) -> ()  [unwired: 9 in, 1 out]
        n61 = event-data("Discard?"=TRUE) -> ()  [unwired: 1 in, 1 out]
      }
      event "Clean 2": Value Change {
        n62 = event-data() -> ()  [unwired: 1 in, 1 out]
        n63 = local read "Pyboard"() -> (w60:string)
        n64 = call "FixCodeSpacing2.vi"("Code"=w60) -> ("Cleaned"=w61:string)  [unwired: 10 in]
        n65 = local write "Pyboard"(w61) -> ()
      }
      event "Run 2": Value Change {
        n66 = event-data() -> ()  [unwired: 1 in, 1 out]
        n67 = call "FixCodeSpacing2.vi"("Code"="Pyboard") -> ("Cleaned"=w62:string)  [unwired: 10 in]
        n68 = local write "Pyboard"(w62) -> ()
        n69 = call "Server_REPL_Script.vi"("Code"=w62, "Server"=w63) -> ()  [unwired: 9 in, 1 out]
      }
      event "Stop 2": Value Change {
        n70 = event-data() -> ()  [unwired: 1 in, 1 out]
        n71 = call "Server_REPL_Abort.vi"("Server"=w65) -> ()  [unwired: 10 in, 1 out]
      }
      event "Save 2": Value Change {
        n72 = event-data() -> ()  [unwired: 1 in, 1 out]
        n73 = local read "Pyboard"() -> (w68:string)
        n74 = call "Server_Save.vi"("Code"=w68, "Name"="Name 2", "Server"=w66) -> ()  [unwired: 8 in, 1 out]
      }
      event "Help 2": Value Change {
        n75 = event-data() -> ()  [unwired: 1 in, 1 out]
        n76 = call "Server_OpenHelp.vi"("Server"=w69) -> ()  [unwired: 10 in, 1 out]
      }
      event "Open Server 2": Value Change {
        n77 = event-data() -> ()  [unwired: 1 in, 1 out]
        n78 = call "Server_OpenServer.vi"("Server"=w70) -> ()  [unwired: 10 in, 1 out]
      }
      event "Files 2": Value Change {
        n79 = event-data() -> ()  [unwired: 1 in, 1 out]
        n80 = call "SpawnProgram.vi"("Server"=w72, "Dialog"=enum16{"Help", "Files"}."Files") -> ()  [unwired: 10 in]
      }
      event Panel Close? {
        w73 = TRUE ("Discard?")
        n81 = event-data() -> ()  [unwired: 1 in, 1 out]
        n82 = event-data("Discard?"=w73) -> ()  [unwired: 1 in, 1 out]
      }
    }
  }
  n83 = call "SetCodePreferences.vi"("Color choices"=T1 {"Quote"=46086, "Comment"=15665920, "Python"=14453248, "Text"=0, "Triple Quote"=9306312, "function"=239, "Line numbers"=9306312, "REPL Err"=15665920, "REPL Text"=0, "Text Bkgd"=16777215, "REPL Bkgd"=16777215}) -> ()  [unwired: 11 in]
